vi "Ora sotto data.vi"(11 "Array in":string[][](array[string])) -> (3 "Array out":string[][](array[string]))   [LabVIEW 2019]
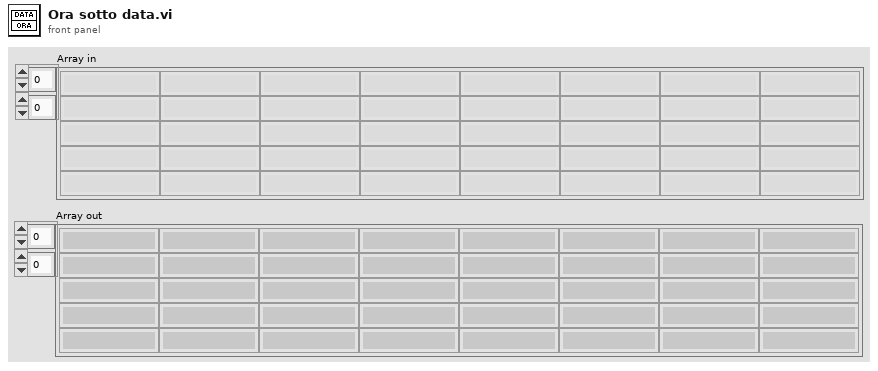
[diagram p1: front panel]
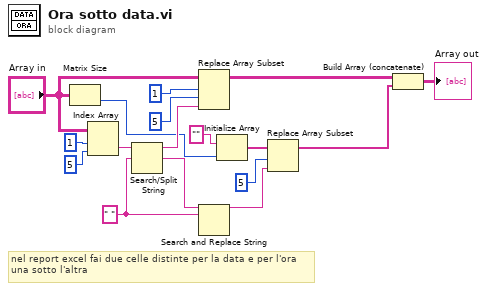
[diagram p0: block diagram]
diagram:
  w9 = " " ("search string/char (-)")
  # "nel report excel fai due celle distinte per la data e per l'ora\nuna sotto l'altra"
  n1 = Matrix Size(0:"Array in") -> (2:w1:i32)  [unwired: 1 out]
  n2 = Index Array(array="Array in", index (row)=1, index (col)=5 ("disabled index (col)")) -> (element=w4:string)
  n3 = Search/Split String(string=w4, search string/char (-)=w9) -> (substring before match=w7:string, match + rest of string=w8:string)  [unwired: 1 in, 1 out]
  n4 = Replace Array Subset(array="Array in", new element=w7, index (row)=1, index (col)=5 ("disabled index (col)")) -> (w15:string[][])
  n5 = Search and Replace String(input string=w8, search string=w9) -> (result string=w14:string)  [unwired: 6 in, 3 out]
  n6 = Initialize Array("", w1) -> (w12:string[])
  n7 = Replace Array Subset "Replace Array Subset"(array=w12, new element=w14, index=5) -> (w16:string[])
  n8 = Build Array (concatenate)(w15, w16) -> (→"Array out":string[][])
